vi "Clear Array.vi"(6 "Variant in":variant, 7 "Shift Pressed?":bool, 8 "error in (no error)":errorcluster, 10 "QD Combo Box Ref":refnum<vi>, 11 "QD Launch VI Ref":refnum<vi>) -> (0 "error out":errorcluster, 4 "Variant out":variant)   [LabVIEW 2014, in "Clear Array.lvlib"]
doc: "Clears the selected array(s) and sets the default value to empty. If shift is also pressed while viewing the front panel, it will affect all front panel arrays, regardless of selection. \n\nDefault Shortcut - [C]"
uses:
  Clear Array.lvlib
panel:
  # "Do not change the connector pane of this VI.\n\nSee the block diagram for directions on how to use this template."
  # "Specify the name of the Undo transaction"
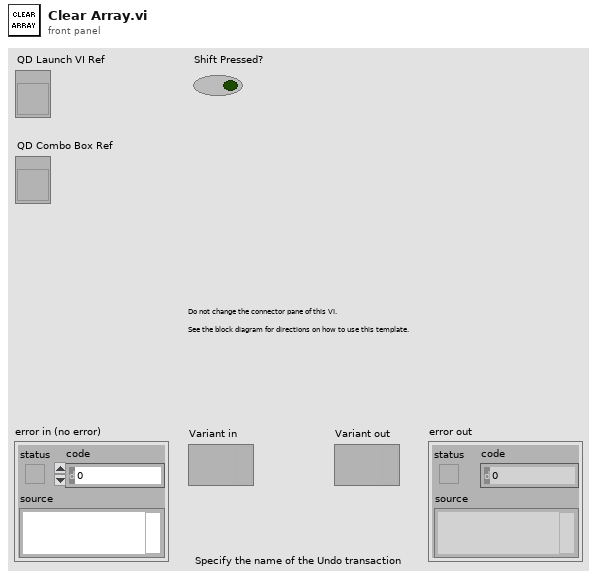
[diagram p1: front panel]
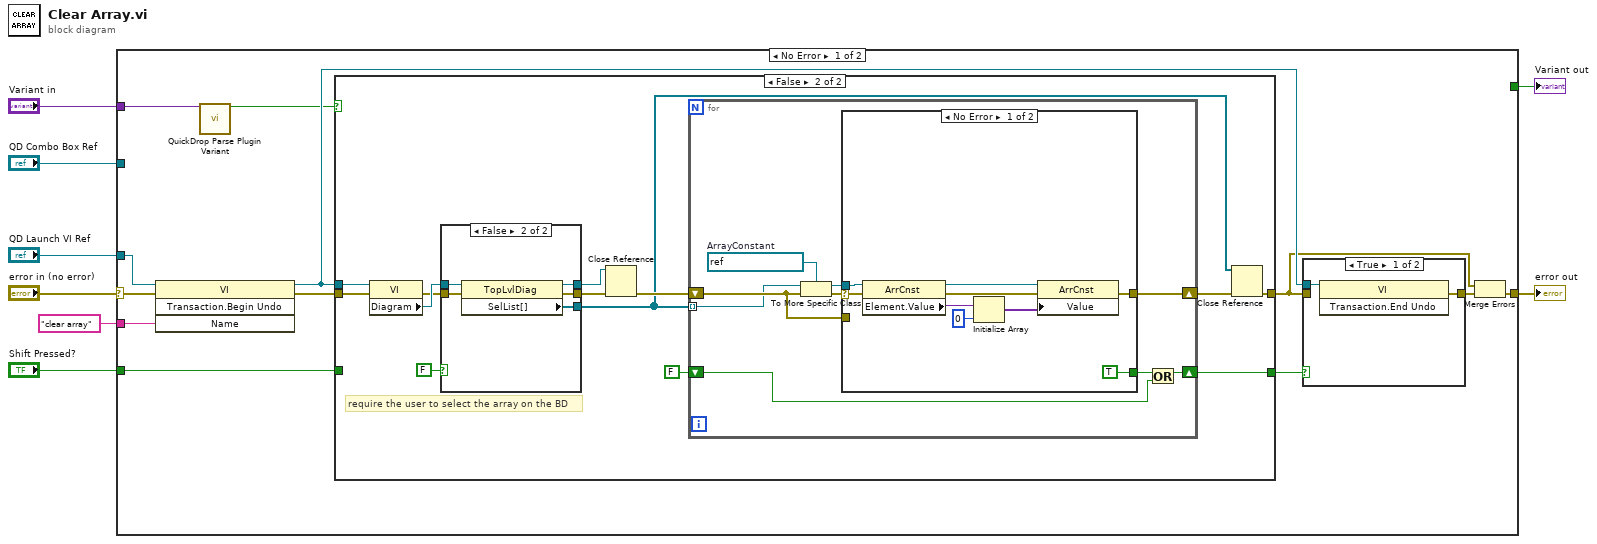
[diagram p0: block diagram]
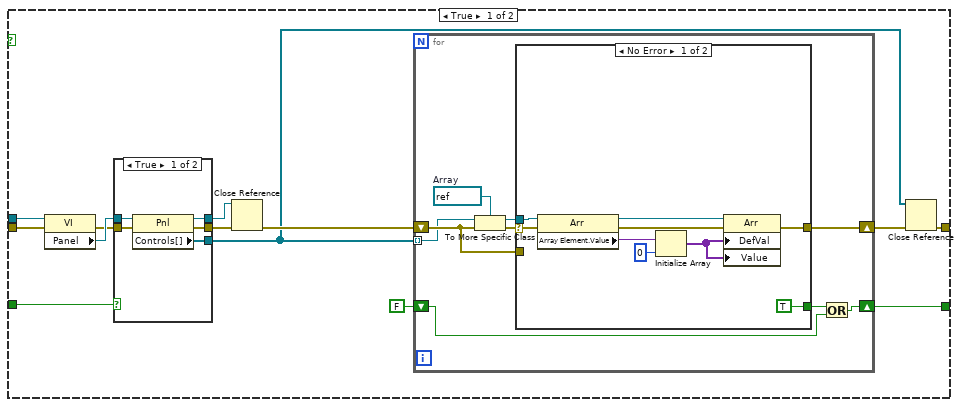
[diagram p2: hidden frame]
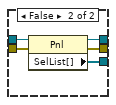
[diagram p3: hidden frame]
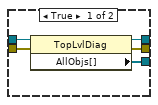
[diagram p5: hidden frame]
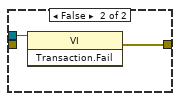
[diagram p7: hidden frame]
diagram:
  n1 = case shown="No Error" "error in (no error)" {
    selector: "error in (no error)" -> [w20 w110]
    tunnel: [w10 w110] -> w7
    tunnel: "QD Launch VI Ref" -> [w19 _]
    tunnel: "Shift Pressed?" -> [w14 _]
    tunnel: "QD Combo Box Ref" -> [_ _]
    tunnel: "Variant in" -> [w21 _]
    tunnel: "clear array" ("Undo Name") -> [w18 _]
    tunnel: [TRUE _] -> w1
    frame No Error {
      n2 = invoke class="VI" method="Transaction.Begin Undo"(reference=w19, error in=w20, "Name"=w18) -> (reference out=w13:refnum<vi>, error out=w16:errorcluster)  [unwired: 1 in, 2 out]
      n3 = call <vilib>:"QuickDrop Parse Plugin Variant.vi"("QDKS Variant in"=w21) -> ("QD Launch VI Panel?"=w12:bool)  [unwired: 12 in, 2 out]
      n4 = case shown="False" w12 {
        tunnel: w16 -> [w34 w76]
        tunnel: [w30 w72] -> w9
        tunnel: w14 -> [w25 _]
        tunnel: w13 -> [w28 w70]
        tunnel: [w23 w66] -> w11
        frame True {
          n5 = property class="VI"(reference=w28, error in=w34) -> (error out=w26:errorcluster, "Panel"=w27:refnum<vi>)  [unwired: 1 out]
          n6 = case shown="True" w25 {
            tunnel: [w39 w44] -> w32
            tunnel: [w38 w43] -> w31
            tunnel: [w37 w42] -> w29
            tunnel: w27 -> [w36 w41]
            tunnel: w26 -> [w35 w40]
            frame True {
              n7 = property class="Pnl"(reference=w36, error in=w35) -> (reference out=w38:refnum<vi>, error out=w39:errorcluster, "Controls[]"=w37:refnum<vi>[])
            }
            frame False {
              n8 = property class="Pnl"(reference=w41, error in=w40) -> (reference out=w43:refnum<vi>, error out=w44:errorcluster, "SelList[]"=w42:refnum<vi>[])
            }
          }
          n9 = Close Reference(reference=w31, error in (no error)=w32) -> (error out=w33:errorcluster)
          n10 = for {
            shift-right: [w53] -> w24
            shift-left: w33 -> [w50]
            tunnel: w29 -> [w49] mode=indexing
            shift-right: [w46] -> w23
            shift-left: FALSE -> [w45]
            w48 = refnum<vi> refnum  # Array
            n11 = To More Specific Class(target class=w48, reference=w49, error in=w50) -> (specific class reference=w52:refnum<vi>, error out=w51:errorcluster)
            n12 = case shown="No Error" w51 {
              selector: w51 -> [w57 _]
              tunnel: [w56 w63] -> w53
              tunnel: w52 -> [w58 _]
              tunnel: w50 -> [_ w63]
              tunnel: [TRUE _] -> w47
              frame No Error {
                n13 = property class="Arr"(reference=w58, error in=w57) -> (reference out=w61:refnum<vi>, error out=w62:errorcluster, "Array Element.Value"=w60:variant)
                n14 = Initialize Array(w60, 0 ("dimension size")) -> (w55:variant[])
                n15 = property class="Arr"(reference=w61, error in=w62, "DefVal"=w55, "Value"=w55) -> (error out=w56:errorcluster)  [unwired: 1 out]
              }
              frame Error {
              }
            }
            n16 = Or(x=w47, y=w45) -> (x .or. y?=w46:bool)
          }
          n17 = Close Reference(reference=w29, error in (no error)=w24) -> (error out=w30:errorcluster)
        }
        frame False {
          # "require the user to select the array on the BD"
          n18 = property class="VI"(reference=w70, error in=w76) -> (error out=w68:errorcluster, "Diagram"=w69:refnum<vi>)  [unwired: 1 out]
          n19 = case shown="False" FALSE {
            tunnel: [w81 w86] -> w74
            tunnel: [w80 w85] -> w73
            tunnel: [w79 w84] -> w71
            tunnel: w69 -> [w78 w83]
            tunnel: w68 -> [w77 w82]
            frame True {
              n20 = property class="TopLvlDiag"(reference=w78, error in=w77) -> (reference out=w80:refnum<vi>, error out=w81:errorcluster, "AllObjs[]"=w79:refnum<vi>[])
            }
            frame False {
              n21 = property class="TopLvlDiag"(reference=w83, error in=w82) -> (reference out=w85:refnum<vi>, error out=w86:errorcluster, "SelList[]"=w84:refnum<vi>[])
            }
          }
          n22 = Close Reference(reference=w73, error in (no error)=w74) -> (error out=w75:errorcluster)
          n23 = for {
            shift-right: [w95] -> w67
            shift-left: w75 -> [w92]
            tunnel: w71 -> [w91] mode=indexing
            shift-right: [w88] -> w66
            shift-left: FALSE -> [w87]
            w90 = refnum<vi> refnum  # ArrayConstant
            n24 = To More Specific Class(target class=w90, reference=w91, error in=w92) -> (specific class reference=w94:refnum<vi>, error out=w93:errorcluster)
            n25 = case shown="No Error" w93 {
              selector: w93 -> [w99 _]
              tunnel: [w98 w105] -> w95
              tunnel: w94 -> [w100 _]
              tunnel: w92 -> [_ w105]
              tunnel: [TRUE _] -> w89
              frame No Error {
                n26 = property class="ArrCnst"(reference=w100, error in=w99) -> (reference out=w103:refnum<vi>, error out=w104:errorcluster, "Element.Value"=w102:variant)
                n27 = Initialize Array(w102, 0 ("dimension size")) -> (w96:variant[])
                n28 = property class="ArrCnst"(reference=w103, error in=w104, "Value"=w96) -> (error out=w98:errorcluster)  [unwired: 1 out]
              }
              frame Error {
              }
            }
            n29 = Or(x=w89, y=w87) -> (x .or. y?=w88:bool)
          }
          n30 = Close Reference(reference=w71, error in (no error)=w67) -> (error out=w72:errorcluster)
        }
      }
      n31 = case shown="True" w11 {
        tunnel: w13 -> [w106 w108]
        tunnel: [w107 w109] -> w15
        tunnel: w9 -> [_ _]
        frame True {
          n32 = invoke class="VI" method="Transaction.End Undo"(reference=w106) -> (error out=w107:errorcluster)  [unwired: 2 in, 2 out]
        }
        frame False {
          n33 = invoke class="VI" method="Transaction.Fail"(reference=w108) -> (error out=w109:errorcluster)  [unwired: 2 in, 2 out]
        }
      }
      n34 = Merge Errors(w9, w15) -> (w10:errorcluster)
    }
    frame Error {
    }
  }
  "error out" <- w7
  "Variant out" <- w1
